vi "Diagrama final con subvi simplificados.vi"() -> ()   [LabVIEW 2022 SP3]
uses:
  <vilib>/Instr/_visa.llb/VISA Configure Serial Port (Instr).vi
panel:
  out "x >= y?":bool
  in  "VISA resource name":refnum<visa-resource-name>
  in  "Actualizar direccion":bool
  in  "Configuracion ADS1263":T1 {"Muestras" items=["50", "250", "1000", "2000", "5000", "10000", "15000", "30000"]; "PGA" items=["1", "2", "4", "8", "16", "32"]; "Muestreo" items=["2.5 SPS", "5 SPS", "10 SPS", "16.6 SPS", "20 SPS", "50 SPS", "60 SPS", "100 SPS", "400 SPS", "1200 SPS", "2400 SPS", "4800 SPS", "7200 SPS", "14400 SPS", "19200 SPS", "38400 SPS"]}
  in  "ENVIAR_CONFI":bool
  in  "Direccion":i16=1 min=1 max=127 step=1
  in  "stop":bool
  # "Velocidad de muestreo"
  # "PGA del sistema"
  # "HABILITAR MODO DIFERENCIAL 1 Y 2"
  # "HABILITAR MODO DIFERENCIAL 3 Y 4"
  # "FILTRO PARA AC1 Y AC2"
  # "100Hz"
  # "500Hz"
  # "FILTRO PARA AC3 Y AC4"
  # "100Hz"
  # "500Hz"
  # "MODO DE OPERACION DEMANDA"
  # "MODO DE OPERACION CONTROLADA"
  # "Cantidad de muestras tomadas"
  # "Recibir por LoRa"
  # "Recibir por SD"
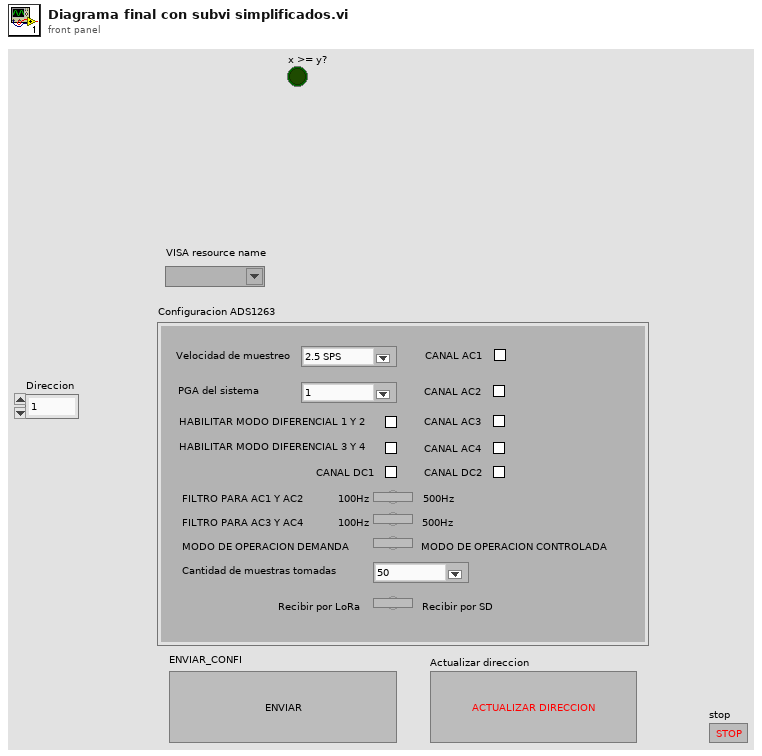
[diagram p1: front panel]
types:
  T1 = cluster{"Muestreo":u32, "PGA":u32, "DIF1Y2":bool, "DIF3Y4":bool, "CANAL AC1":bool, "CANAL AC2":bool, "CANAL AC3":bool, "CANAL AC4":bool, "CANAL DC1":bool, "CANAL DC2":bool, "FILTRO1":bool, "FILTRO2":bool, "MODO OPERACION":bool, "Muestras":u32, "MODO transmision":bool}
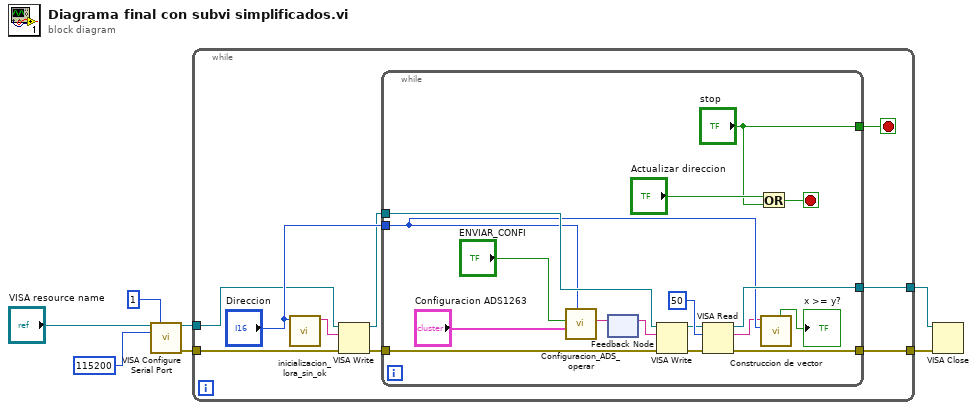
[diagram p0: block diagram]
diagram:
  n1 = call-poly "VISA Configure Serial Port"("VISA resource name"="VISA resource name", "timeout (10sec)"=u32 1, "baud rate (9600)"=u32 115200) -> ("VISA resource name out"=w4:refnum<visa-resource-name>, "error out"=w3:errorcluster)  [unwired: 11 in]
  n2 = while {
    tunnel: w4 -> [w15]
    tunnel: w3 -> [w14]
    tunnel: [w9] -> w2
    tunnel: [w8] -> w1
    stop <- w10 stop-if-true
    n3 = call "inicializacion_lora_sin_ok.vi"("Direccion"="Direccion") -> ("concatenated string 2"=w13:string)  [unwired: 10 in]
    n4 = VISA Write(VISA resource name=w15, write buffer=w13, error in (no error)=w14) -> (VISA resource name out=w12:refnum<visa-resource-name>, error out=w11:errorcluster)  [unwired: 1 out]
    n5 = while {
      tunnel: "Direccion" -> [w19]
      tunnel: w12 -> [w25]
      tunnel: w11 -> [w24]
      tunnel: ["stop"] -> w10
      tunnel: [w27] -> w9
      tunnel: [w26] -> w8
      stop <- w30 stop-if-true
      n6 = call "Configuracion_ADS_operar.vi"("Direccion"=w19, "Configuracion ADS1263"="Configuracion ADS1263", "ENVIAR_CONFI"="ENVIAR_CONFI") -> ("Configuracion"=w21:string)  [unwired: 7 in, 1 out]
      n7 = feedback-in #1(w21) -> ()
      n8 = feedback #1() -> (w20:string)  [unwired: 1 in]
      n9 = VISA Write(VISA resource name=w25, write buffer=w20, error in (no error)=w24) -> (VISA resource name out=w23:refnum<visa-resource-name>, error out=w22:errorcluster)  [unwired: 1 out]
      n10 = VISA Read(VISA resource name=w23, byte count=u32 50, error in (no error)=w22) -> (VISA resource name out=w27:refnum<visa-resource-name>, read buffer=w18:string, error out=w26:errorcluster)  [unwired: 1 out]
      n11 = Or(x="Actualizar direccion", y="stop") -> (x .or. y?=w30:bool)
      n12 = call "Construccion de vector.vi"("Direccion"=w19, "Leer puerto"=w18) -> ("x >= y?"=→"x >= y?":bool)  [unwired: 9 in]
    }
  }
  n13 = VISA Close(VISA resource name=w2, error in (no error)=w1) -> ()  [unwired: 1 out]
